vi "LockServoWhileMoving.vi"(11 "Connection Cluster in":T1) -> (3 "Connection Cluster out 2":T1)   [LabVIEW 2013]
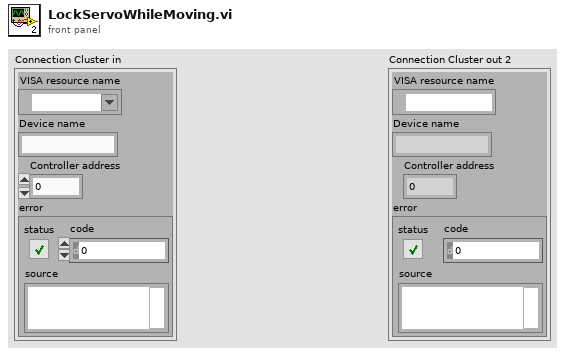
[diagram p1: front panel]
types:
  T1 = cluster{"VISA resource name":refnum<visa-resource-name>, "Device name":string, "Controller address":i32, "error":errorcluster}
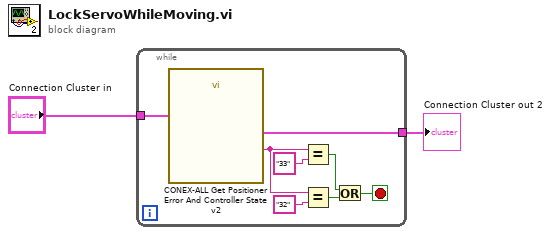
[diagram p0: block diagram]
diagram:
  n1 = while {
    tunnel: "Connection Cluster in" -> [w10]
    tunnel: [w9] -> w1
    stop <- w6 stop-if-true
    n2 = call <userlib>:"CONEX-ALL Get Positioner Error And Controller State v2.vi"("Connection Cluster in"=w10) -> ("Controller state"=w4:string, "Connection Cluster out"=w9:T1)  [unwired: 8 in, 1 out]
    n3 = Equal?(x=w4, y="33") -> (x = y?=w7:bool)
    n4 = Equal?(x=w4, y="32") -> (x = y?=w5:bool)
    n5 = Or(x=w7, y=w5) -> (x .or. y?=w6:bool)
  }
  "Connection Cluster out 2" <- w1
